vi "String.Generate Str ID from Time Secs.vi"(10 "FracSec Len":i32=3, 11 "Sec Len":i32=6) -> (3 "ID":string)   [LabVIEW 2019]
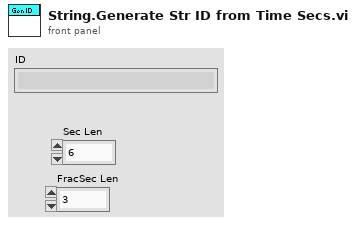
[diagram p1: front panel]
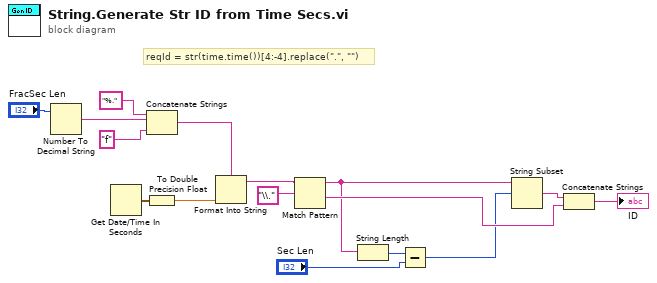
[diagram p0: block diagram]
diagram:
  # "reqId = str(time.time())[4:-4].replace(\".\", \"\")"
  n1 = Number To Decimal String(number="FracSec Len") -> (decimal integer string=w3:string)  [unwired: 1 in]
  n2 = Get Date/Time In Seconds() -> (seconds since 1Jan1904=w1:timestamp)
  n3 = Concatenate Strings("%." ("format string"), w3, "f" ("format string")) -> (w2:string)
  n4 = To Double Precision Float(number=w1) -> (double precision float=w11:dbl)
  n5 = Format Into String(format string=w2, w11) -> (resulting string=w16:string)  [unwired: 2 in, 1 out]
  n6 = Match Pattern(string=w16, regular expression="\\.") -> (before substring=w10:string, after substring=w13:string)  [unwired: 1 in, 2 out]
  n7 = String Length(string=w10) -> (length=w9:i32)
  n8 = Subtract(x=w9, y="Sec Len") -> (x-y=w7:i32)
  n9 = String Subset(string=w10, offset (0)=w7) -> (substring=w14:string)  [unwired: 1 in]
  n10 = Concatenate Strings(w14, w13) -> (→"ID":string)
